vi "Exercise 4.4 RPi Cam to JPG.vi"() -> ()   [LabVIEW 2014]
uses:
  <vilib>/Q-Wave Systems/QwaveSys RPi Training Package (Demo)/Addons/QwaveSys RPi Training Library.lvlib
panel:
  in  "File Path":string="/home/pi/cam0.jpg"
  out "standard output":string
  out "Cmd":string
  out "Output 2":picture
  in  "Image Size":T1(ring)
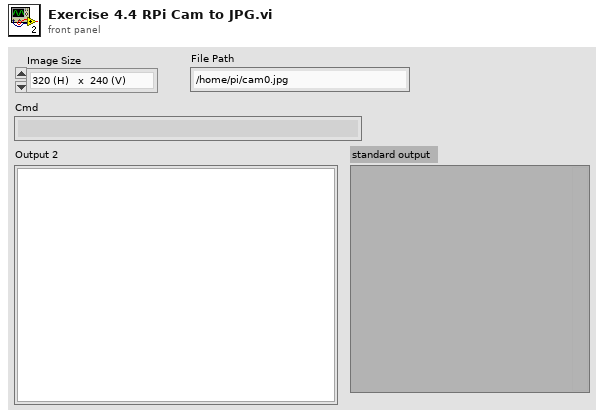
[diagram p1: front panel]
types:
  T1 = enum16{"320 (H)   x  240 (V)", "352(H)    x  288 (V)", "640 (H)   x  480 (V) ", "800 (H)   x  600 (V)", "1024 (H) x  768 (V)", "1280 (H) x  720 (V)", "1280 (H) x 1024 (V)", "1920 (H) x 1080 (V)"}
  T2 = typedef "imagedata.ctl" = cluster{"image type":i32, "image depth":i32, "image":u8[], "mask":u8[], "colors":u32[], "Rectangle":cluster{"left":i16, "top":i16, "right":i16, "bottom":i16}}
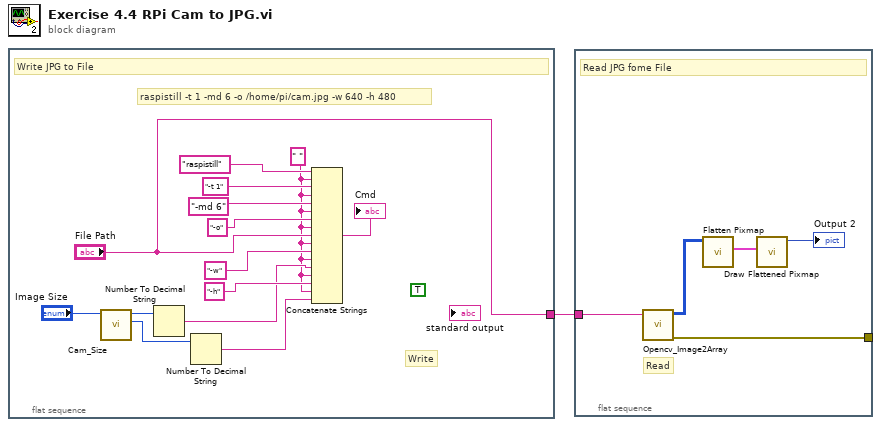
[diagram p0: block diagram]
diagram:
  n1 = flat-sequence {
    tunnel: ["File Path"] -> w1
    frame #0 {
      (unwired) TRUE ("wait until completion? (T)")
      w2 = " "
      # "Write"
      # "raspistill -t 1 -md 6 -o /home/pi/cam.jpg -w 640 -h 480"
      # "Write JPG to File"
      n2 = call <vilib>:"Cam_Size.vi"("Image Size"="Image Size") -> ("h"=w13:i32, "w"=w14:i32)  [unwired: 8 in, 1 out]
      n3 = Number To Decimal String(number=w14) -> (decimal integer string=w6:string)  [unwired: 1 in]
      n4 = Number To Decimal String(number=w13) -> (decimal integer string=w3:string)  [unwired: 1 in]
      n5 = Concatenate Strings("raspistill", w2, "-t 1", w2, "-md 6", w2, "-o", w2, "File Path", w2, "-w", w2, w6, w2, "-h", w2, w3) -> (→"Cmd":string)
    }
  }
  n6 = flat-sequence {
    tunnel: [w17] -> _
    tunnel: w1 -> [w16]
    frame #0 {
      # "Read"
      # "Read JPG fome File"
      n7 = call <vilib>:"Opencv_Image2Array.vi"("filename"=w16) -> ("error out"=w17:errorcluster, "Image Pixels 24 bits"=w18:u32[][])  [unwired: 8 in, 1 out]
      n8 = call <vilib>:"Flatten Pixmap.vi"("24-bit pixmap"=w18) -> ("image data"=w19:T2)  [unwired: 10 in]
      n9 = call <vilib>:"Draw Flattened Pixmap.vi"("image data"=w19) -> ("new picture"=→"Output 2":picture)  [unwired: 8 in]
    }
  }
